vi "VI Tree.vi"   [LabVIEW 2021, in "Yokogawa WT1800 Series.lvlib"]
doc: "This is the instrument driver for the Yokogawa WT1800 Series Digital Power Meter. The VI Tree displays all the user-callable VIs of the instrument driver in an organized table."
uses:
  <instrlib>/Yokogawa WT1800 Series/Yokogawa WT1800 Series.lvlib
  <instrlib>/Yokogawa WT1800 Series/Public/Configure/Configure Range (Voltage).vi
  <instrlib>/Yokogawa WT1800 Series/Public/Configure/Configure Motor (Analog Speed).vi
  <instrlib>/Yokogawa WT1800 Series/Public/Configure/Configure Filter (Line).vi
  <instrlib>/Yokogawa WT1800 Series/Public/Configure/Configure User Defined Event (Range).vi
  <instrlib>/Yokogawa WT1800 Series/Public/Action-Status/Query Numeric (Normal).vi
  <instrlib>/Yokogawa WT1800 Series/Public/Data/Read Waveform (Single).vi
  <instrlib>/Yokogawa WT1800 Series/Public/Data/Read Measurement (Normal).vi
  <instrlib>/Yokogawa WT1800 Series/Public/Data/Low Level/Fetch Measurement (Normal).vi
  <instrlib>/Yokogawa WT1800 Series/Public/Utility/Function/Create Function String (Voltage).vi
panel:
  # "(c) 2011 Yokogawa Meters & Instruments.  All rights reserved."
  # "SEE DIAGRAM\nFOR VI TREE."
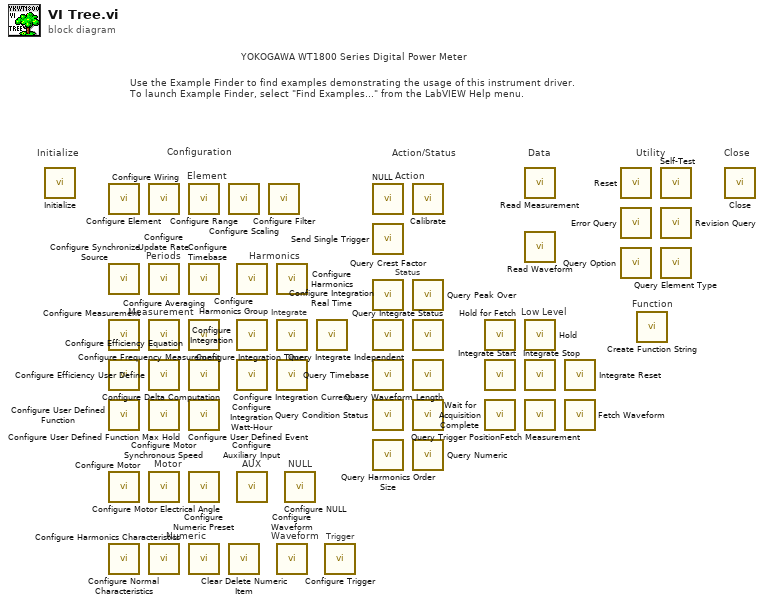
[diagram p0: block diagram]
diagram:
  # "Low Level"
  # "Waveform"
  # "Numeric"
  # "NULL"
  # "Status"
  # "Action"
  # "AUX"
  # "Trigger"
  # "Motor"
  # "Harmonics"
  # "Integrate"
  # "Function"
  # "Measurement"
  # "Periods"
  # "Element"
  # "YOKOGAWA WT1800 Series Digital Power Meter"
  # "Use the Example Finder to find examples demonstrating the usage of this instrument driver.\nTo launch Example Finder, select \"Find Examples...\" from the LabVIEW Help menu."
  # "Configuration"
  # "Utility"
  # "Data"
  # "Action/Status"
  # "Close"
  # "Initialize"
  n1 = call <instrlib>:"Initialize.vi"() -> ()  [unwired: 10 in, 2 out]
  n2 = call <instrlib>:"Configure Element.vi"() -> ()  [unwired: 10 in, 2 out]
  n3 = call <instrlib>:"Configure Synchronize Source.vi"() -> ()  [unwired: 10 in, 2 out]
  n4 = call <instrlib>:"Configure Measurement.vi"() -> ()  [unwired: 14 in, 2 out]
  n5 = call <instrlib>:"Configure Efficiency Equation.vi"() -> ()  [unwired: 10 in, 2 out]
  n6 = call <instrlib>:"Configure User Defined Function.vi"() -> ()  [unwired: 10 in, 2 out]
  n7 = call-poly <instrlib>:"Configure Motor.vi"() -> ()  [unwired: 14 in, 2 out]
  n8 = call <instrlib>:"Configure Normal Characteristics.vi"() -> ()  [unwired: 10 in, 2 out]
  n9 = call <instrlib>:"Configure Wiring.vi"() -> ()  [unwired: 14 in, 2 out]
  n10 = call <instrlib>:"Configure Update Rate.vi"() -> ()  [unwired: 10 in, 2 out]
  n11 = call <instrlib>:"Configure Averaging.vi"() -> ()  [unwired: 10 in, 2 out]
  n12 = call <instrlib>:"Configure Efficiency User Define.vi"() -> ()  [unwired: 10 in, 2 out]
  n13 = call <instrlib>:"Configure User Defined Function Max Hold.vi"() -> ()  [unwired: 10 in, 2 out]
  n14 = call <instrlib>:"Configure Motor Synchronous Speed.vi"() -> ()  [unwired: 14 in, 2 out]
  n15 = call <instrlib>:"Configure Harmonics Characteristics.vi"() -> ()  [unwired: 10 in, 2 out]
  n16 = call-poly <instrlib>:"Configure Range.vi"() -> ()  [unwired: 14 in, 2 out]
  n17 = call <instrlib>:"Configure Timebase.vi"() -> ()  [unwired: 10 in, 2 out]
  n18 = call <instrlib>:"Configure Frequency Measurement.vi"() -> ()  [unwired: 10 in, 2 out]
  n19 = call <instrlib>:"Configure Delta Computation.vi"() -> ()  [unwired: 10 in, 2 out]
  n20 = call-poly <instrlib>:"Configure User Defined Event.vi"() -> ()  [unwired: 14 in, 2 out]
  n21 = call <instrlib>:"Configure Motor Electrical Angle.vi"() -> ()  [unwired: 10 in, 2 out]
  n22 = call <instrlib>:"Configure Numeric Preset.vi"() -> ()  [unwired: 10 in, 2 out]
  n23 = call <instrlib>:"Configure Scaling.vi"() -> ()  [unwired: 14 in, 2 out]
  n24 = call <instrlib>:"Clear Delete Numeric Item.vi"() -> ()  [unwired: 10 in, 2 out]
  n25 = call <instrlib>:"Configure Harmonics Group.vi"() -> ()  [unwired: 10 in, 2 out]
  n26 = call <instrlib>:"Configure Integration.vi"() -> ()  [unwired: 10 in, 2 out]
  n27 = call <instrlib>:"Configure Integration Watt-Hour.vi"() -> ()  [unwired: 10 in, 2 out]
  n28 = call <instrlib>:"Configure Auxiliary Input.vi"() -> ()  [unwired: 14 in, 2 out]
  n29 = call-poly <instrlib>:"Configure Filter.vi"() -> ()  [unwired: 10 in, 2 out]
  n30 = call <instrlib>:"Configure Harmonics.vi"() -> ()  [unwired: 14 in, 2 out]
  n31 = call <instrlib>:"Configure Integration Timer.vi"() -> ()  [unwired: 10 in, 2 out]
  n32 = call <instrlib>:"Configure Integration Current.vi"() -> ()  [unwired: 10 in, 2 out]
  n33 = call <instrlib>:"Configure Waveform.vi"() -> ()  [unwired: 10 in, 2 out]
  n34 = call <instrlib>:"Configure NULL.vi"() -> ()  [unwired: 10 in, 2 out]
  n35 = call <instrlib>:"Configure Integration Real Time.vi"() -> ()  [unwired: 14 in, 2 out]
  n36 = call <instrlib>:"Configure Trigger.vi"() -> ()  [unwired: 10 in, 2 out]
  n37 = call <instrlib>:"NULL.vi"() -> ()  [unwired: 10 in, 2 out]
  n38 = call <instrlib>:"Send Single Trigger.vi"() -> ()  [unwired: 10 in, 2 out]
  n39 = call <instrlib>:"Query Crest Factor.vi"() -> ()  [unwired: 9 in, 3 out]
  n40 = call <instrlib>:"Query Integrate Independent.vi"() -> ()  [unwired: 9 in, 3 out]
  n41 = call <instrlib>:"Query Timebase.vi"() -> ()  [unwired: 9 in, 3 out]
  n42 = call <instrlib>:"Query Condition Status.vi"() -> ()  [unwired: 9 in, 3 out]
  n43 = call <instrlib>:"Query Harmonics Order Size.vi"() -> ()  [unwired: 9 in, 3 out]
  n44 = call <instrlib>:"Calibrate.vi"() -> ()  [unwired: 9 in, 3 out]
  n45 = call <instrlib>:"Query Peak Over.vi"() -> ()  [unwired: 8 in, 4 out]
  n46 = call <instrlib>:"Query Integrate Status.vi"() -> ()  [unwired: 8 in, 4 out]
  n47 = call <instrlib>:"Query Waveform Length.vi"() -> ()  [unwired: 9 in, 3 out]
  n48 = call <instrlib>:"Query Trigger Position.vi"() -> ()  [unwired: 9 in, 3 out]
  n49 = call-poly <instrlib>:"Query Numeric.vi"() -> ()  [unwired: 9 in, 3 out]
  n50 = call <instrlib>:"Hold for Fetch.vi"() -> ()  [unwired: 10 in, 2 out]
  n51 = call <instrlib>:"Integrate Start.vi"() -> ()  [unwired: 10 in, 2 out]
  n52 = call <instrlib>:"Wait for Acquisition Complete.vi"() -> ()  [unwired: 10 in, 2 out]
  n53 = call-poly <instrlib>:"Read Measurement.vi"() -> ()  [unwired: 8 in, 4 out]
  n54 = call-poly <instrlib>:"Read Waveform.vi"() -> ()  [unwired: 9 in, 3 out]
  n55 = call <instrlib>:"Hold.vi"() -> ()  [unwired: 10 in, 2 out]
  n56 = call <instrlib>:"Integrate Stop.vi"() -> ()  [unwired: 10 in, 2 out]
  n57 = call-poly <instrlib>:"Fetch Measurement.vi"() -> ()  [unwired: 8 in, 4 out]
  n58 = call <instrlib>:"Integrate Reset.vi"() -> ()  [unwired: 10 in, 2 out]
  n59 = call <instrlib>:"Fetch Waveform.vi"() -> ()  [unwired: 9 in, 3 out]
  n60 = call <instrlib>:"Reset.vi"() -> ()  [unwired: 10 in, 2 out]
  n61 = call <instrlib>:"Error Query.vi"() -> ()  [unwired: 8 in, 4 out]
  n62 = call <instrlib>:"Query Option.vi"() -> ()  [unwired: 13 in, 3 out]
  n63 = call-poly <instrlib>:"Create Function String.vi"() -> ()  [unwired: 9 in, 3 out]
  n64 = call <instrlib>:"Self-Test.vi"() -> ()  [unwired: 8 in, 4 out]
  n65 = call <instrlib>:"Revision Query.vi"() -> ()  [unwired: 8 in, 4 out]
  n66 = call <instrlib>:"Query Element Type.vi"() -> ()  [unwired: 9 in, 3 out]
  n67 = call <instrlib>:"Close.vi"() -> ()  [unwired: 11 in, 1 out]
